vi "Recieve Response with Result.vi"(4 "Finished":bool=TRUE, 6 "Result":refnum<class "Mag Lab Result.lvclass">, 8 "error in (no error)":errorcluster, 9 "Requestor":string, 10 "Requestee":string, 11 "Common Measurements in":refnum<class "Common Measurements.lvclass">) -> (0 "error out":errorcluster, 3 "Common Measurements out":refnum<class "Common Measurements.lvclass">)   [LabVIEW 2015, in "Common Measurements.lvclass"]
uses:
  Common Measurements.lvclass
  Mag Lab Result/Mag Lab Result.lvclass
  Mag Lab Result/Mag Lab Result.lvclass/Mag Lab Result.ctl
  Mag Lab Measure Base/Mag Lab Measure Base.lvclass/Mag Lab Measure Base.ctl
  Common Measurements Interface Messages/Update time Msg/Update time Msg.lvclass/Update time Msg.ctl
  <vilib>/ActorFramework/Message Enqueuer/Message Enqueuer.lvclass/Message Enqueuer.ctl
  <vilib>/ActorFramework/Message Enqueuer/Enqueue.vi
  <vilib>/ActorFramework/Message Priority Queue/Priority Enqueue.vi
  Mag Lab Measure Controller/Mag Lab Measure Controller.lvclass
  <vilib>/ActorFramework/Message Enqueuer/Message Enqueuer.lvclass
  Common Measurements Interface Messages/Update time Msg/Update time Msg.lvclass
  Mag Lab Measure Base/Mag Lab Measure Base.lvclass
  Mag Lab Error Handler/Mag Lab Error Handler.lvclass
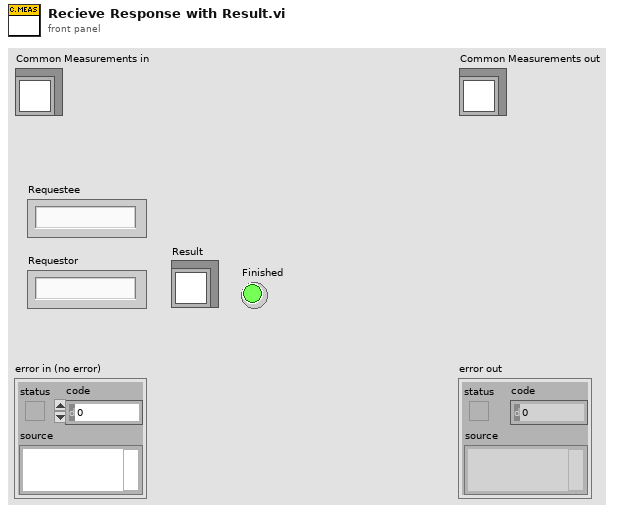
[diagram p1: front panel]
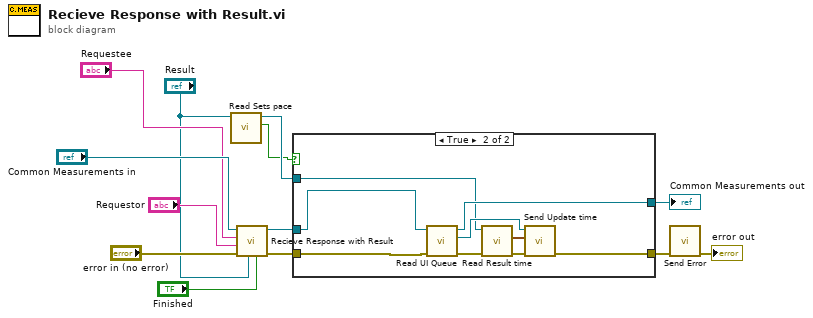
[diagram p0: block diagram]
diagram:
  n1 = call "Read Sets pace.vi"("Mag Lab Result in"="Result") -> ("Sets pace"=w1:bool, "Mag Lab Result out"=w2:refnum<class "Mag Lab Result.lvclass">)  [unwired: 8 in, 1 out]
  n2 = call-parent "Recieve Response with Result.vi"("Finished"="Finished", "Result"="Result", "error in (no error)"="error in (no error)", "Requestor"="Requestor", "Requestee"="Requestee", "Mag Lab Measure Controller in"="Common Measurements in") -> ("error out"=w5:errorcluster, "Mag Lab Measure Controller out"=w8:refnum<class "Common Measurements.lvclass">)  [unwired: 4 in]
  n3 = case shown="True" w1 {
    tunnel: w8 -> [w15 w24]
    tunnel: [w15 w23] -> w7
    tunnel: w2 -> [_ w16]
    tunnel: w5 -> [w14 w17]
    tunnel: [w14 w18] -> w3
    frame False {
    }
    frame True {
      n4 = call "Read UI Queue.vi"("error in (no error)"=w17, "Mag Lab Measure Base in"=w24) -> ("error out"=w22:errorcluster, "Actor Framework.lvlib:Message Enqueuer"=w21:refnum<class "Message Enqueuer.lvclass">, "Mag Lab Measure Base out"=w23:refnum<class "Common Measurements.lvclass">)  [unwired: 7 in]
      n5 = call "Read Result time.vi"("error in (no error)"=w22, "Mag Lab Result in"=w16) -> ("error out"=w20:errorcluster, "Result time"=w19:timestamp)  [unwired: 7 in, 1 out]
      n6 = call "Send Update time.vi"("error in (no error)"=w20, "Time Stamp Control"=w19, "Message Enqueuer"=w21) -> ("error out"=w18:errorcluster)  [unwired: 7 in, 1 out]
    }
  }
  "Common Measurements out" <- w7
  n7 = call "Send Error.vi"("error in (no error)"=w3) -> ("error out"=→"error out":errorcluster)  [unwired: 9 in, 1 out]
